vi "Instantaneous COR.vi"(1 "Data Input":T1 {"Data Channels" format="%.2f"}) -> (0 "Data Output":T1 {"Data Channels" format="%.2f"})   [LabVIEW 2013]
uses:
  <vilib>/Analysis/baseanly.llb/Real A x B.vi
  <vilib>/Analysis/baseanly.llb/Real Inverse Matrix.vi
  comm/fick-matrix/fick-matrix.lvlib
  <vilib>/Analysis/NI_AALBase.lvlib
panel:
  in  "Bite-piece channels":cluster{"List 1":u16, "Boolean 2":bool}[](array[cluster])=[{"List 1"=25, "Boolean 2"=TRUE}, {"List 1"=29, "Boolean 2"=FALSE}, {"List 1"=27, "Boolean 2"=FALSE}] {"List 1" items=["Hz Position-in-Head", "Hy Position-in-Head", "Hx Position-in-Head", "Hx Velocity-in-Head", "Hy Velocity-in-Head", "Hz Velocity-in-Head", "Hl Velocity-in-Head", "Hr Velocity-in-Head", "Lz Position-in-Head", "Ly Position-in-Head", "Lx Position-in-Head", "Lx Velocity-in-Head", "Ly Velocity-in-Head", "Lz Velocity-in-Head", "Ll Velocity-in-Head", "Lr Velocity-in-Head", "Rz Position-in-Head", "Ry Position-in-Head", "Rx Position-in-Head", "Rx Velocity-in-Head", "Ry Velocity-in-Head", "Rz Velocity-in-Head", "Rl Velocity-in-Head", "Rr Velocity-in-Head", "Button", "Ascension X", "Ascension X Vel", "Ascension Y", "Ascension Y Vel", "Ascension Z", "Chair Position", "Chair Velocity", " "]}
  in  "Head Channels":cluster{"List 1":u16, "Boolean 2":bool}[](array[cluster])=[{"List 1"=0, "Boolean 2"=FALSE}, {"List 1"=1, "Boolean 2"=FALSE}, {"List 1"=2, "Boolean 2"=FALSE}] {"List 1" items=["Hz Position-in-Head", "Hy Position-in-Head", "Hx Position-in-Head", "Hx Velocity-in-Head", "Hy Velocity-in-Head", "Hz Velocity-in-Head", "Hl Velocity-in-Head", "Hr Velocity-in-Head", "Lz Position-in-Head", "Ly Position-in-Head", "Lx Position-in-Head", "Lx Velocity-in-Head", "Ly Velocity-in-Head", "Lz Velocity-in-Head", "Ll Velocity-in-Head", "Lr Velocity-in-Head", "Rz Position-in-Head", "Ry Position-in-Head", "Rx Position-in-Head", "Rx Velocity-in-Head", "Ry Velocity-in-Head", "Rz Velocity-in-Head", "Rl Velocity-in-Head", "Rr Velocity-in-Head", "Button", "Ascension X", "Ascension X Vel", "Ascension Y", "Ascension Y Vel", "Ascension Z", "Chair Position", "Chair Velocity", " "]}
  # "Inv                 Channel"
  # "Head Z Fick position (deg)\n\nHead Y\n\nHead X"
  # "Inv                 Channel"
  # "Bite-piece X position (mm)\n\nBite-piece Y\n\nBite-piece Z"
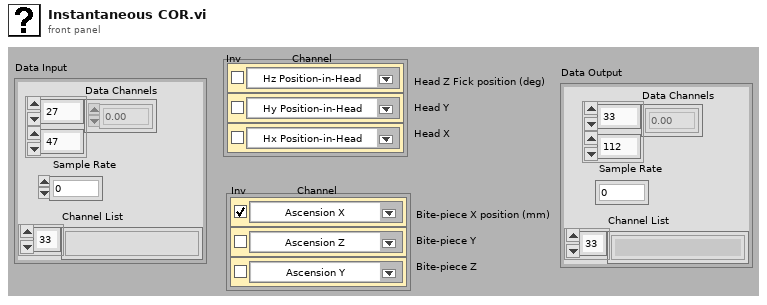
[diagram p1: front panel]
types:
  T1 = cluster{"Data Channels":dbl[][], "Sample Rate":i32, "Channel List":string[]}
  T2 = typedef "NI_Matrix.lvlib/RealMatrix.ctl" = dbl[][]
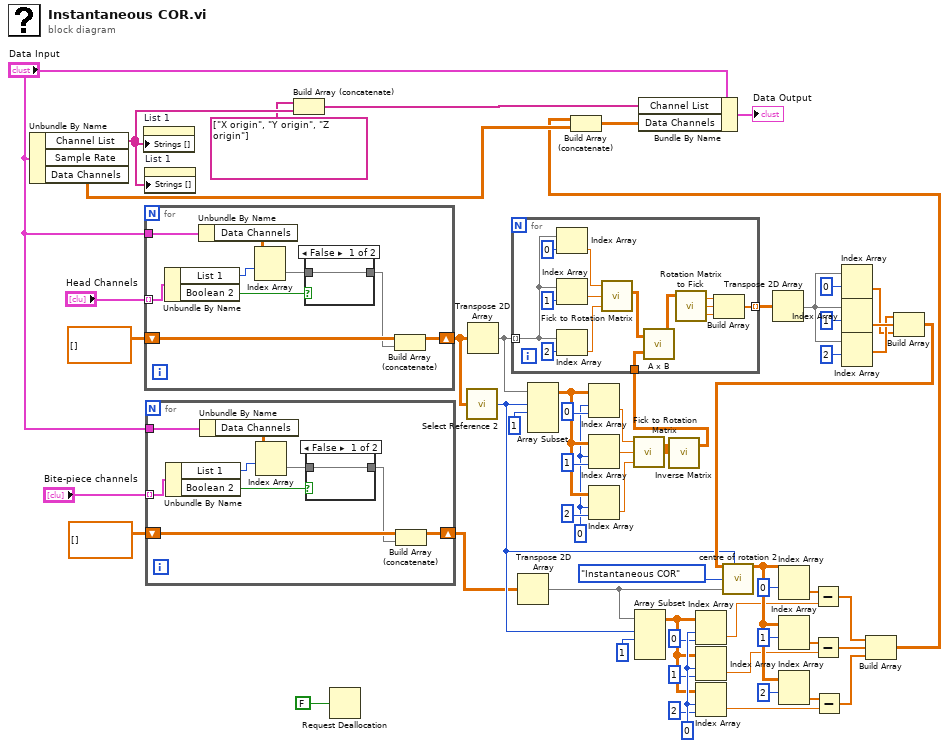
[diagram p0: block diagram]
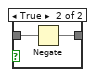
[diagram p2: hidden frame]
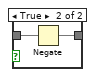
[diagram p3: hidden frame]
diagram:
  w13 = 0 ("disabled index (col)")
  w45 = 0 ("disabled index (col)")
  n1 = Unbundle By Name("Data Input") -> ("Channel List"=w34:string[], "Data Channels"=w35:dbl[][])  [unwired: 1 out]
  n2 = property on="List 1" class="Ring (strict)"("Strings []"=w34) -> ()  [unwired: 2 in, 2 out]
  n3 = property on="List 1" class="Ring (strict)"("Strings []"=w34) -> ()  [unwired: 2 in, 2 out]
  n4 = for {
    tunnel: "Head Channels" -> [w67] mode=indexing
    tunnel: "Data Input" -> [w64]
    shift-right: [w66] -> w37
    shift-left: dbl[][] [] -> [w65]
    n5 = Unbundle By Name(w67) -> ("List 1"=w62:u16, "Boolean 2"=w61:bool)
    n6 = Unbundle By Name(w64) -> ("Data Channels"=w63:dbl[][])
    n7 = Index Array(array=w63, index (row)=w62) -> (element=w60:dbl[])  [unwired: 1 in]
    n8 = case shown="False" w61 {
      tunnel: w60 -> [w68 w70]
      tunnel: [w68 w69] -> w59
      frame False {
      }
      frame True {
        n9 = Negate(x=w70) -> (-x=w69:dbl[])
      }
    }
    n10 = Build Array (concatenate)(w65, w59) -> (w66:dbl[][])
  }
  n11 = for {
    tunnel: "Bite-piece channels" -> [w79] mode=indexing
    tunnel: "Data Input" -> [w76]
    shift-right: [w78] -> w6
    shift-left: dbl[][] [] -> [w77]
    n12 = Unbundle By Name(w79) -> ("List 1"=w74:u16, "Boolean 2"=w73:bool)
    n13 = Unbundle By Name(w76) -> ("Data Channels"=w75:dbl[][])
    n14 = Index Array(array=w75, index (row)=w74) -> (element=w72:dbl[])  [unwired: 1 in]
    n15 = case shown="False" w73 {
      tunnel: w72 -> [w80 w82]
      tunnel: [w80 w81] -> w71
      frame False {
      }
      frame True {
        n16 = Negate(x=w82) -> (-x=w81:dbl[])
      }
    }
    n17 = Build Array (concatenate)(w77, w71) -> (w78:dbl[][])
  }
  n18 = Build Array (concatenate)(string[] ["X origin", "Y origin", "Z origin"], w34) -> (w40:string[])
  n19 = Request Deallocation(FALSE ("flag")) -> ()
  n20 = call "Select Reference 2.vi"("3D Coil"=w37) -> ("Element Data"=w7:i32)
  n21 = Transpose 2D Array(2D array=w37) -> (transposed array=w36:dbl[][])
  n22 = Transpose 2D Array(2D array=w6) -> (transposed array=w2:dbl[][])
  n23 = Array Subset(array=w36, index (row)=w7, length (row)=1 ("length")) -> (w53:dbl[][])  [unwired: 2 in]
  n24 = Index Array(array=w53, index (row)=w45, index (col)=0 ("index (row)")) -> (element=w52:dbl)
  n25 = Index Array(array=w53, index (row)=w45, index (col)=1 ("index (row)")) -> (element=w51:dbl)
  n26 = Index Array(array=w53, index (row)=w45, index (col)=2 ("index (row)")) -> (element=w50:dbl)
  n27 = call "Fick to Rotation Matrix.vi"("T"=w50, "V"=w51, "H"=w52) -> ("Rotation Matrix"=w49:dbl[][])
  n28 = Array Subset(array=w2, index (row)=w7, length (row)=1 ("length")) -> (w9:dbl[][])  [unwired: 2 in]
  n29 = call-poly <vilib>:"Inverse Matrix.vi"("Input Matrix"=w49) -> ("Inverse Matrix"=w44:T2)  [unwired: 1 in, 1 out]
  n30 = for {
    tunnel: w36 -> [w90] mode=indexing
    tunnel: w44 -> [w89]
    tunnel: [w83] -> w43 mode=indexing
    n31 = Index Array(array=w90, index=0 ("index (row)")) -> (element=w94:dbl)
    n32 = Index Array(array=w90, index=1 ("index (row)")) -> (element=w95:dbl)
    n33 = Index Array(array=w90, index=2 ("index (row)")) -> (element=w96:dbl)
    n34 = call "Fick to Rotation Matrix.vi"("T"=w96, "V"=w95, "H"=w94) -> ("Rotation Matrix"=w88:dbl[][])
    n35 = call-poly <vilib>:"A x B.vi"("B"=w89, "A"=w88) -> ("A x B"=w87:T2)  [unwired: 1 out]
    n36 = call "Rotation Matrix to Fick.vi"("A"=w87) -> ("T"=w84:dbl, "V"=w85:dbl, "H"=w86:dbl)  [unwired: 2 in]
    n37 = Build Array(w86, w85, w84) -> (w83:dbl[])
  }
  n38 = Index Array(array=w9, index (row)=w13, index (col)=0 ("index (row)")) -> (element=w5:dbl)
  n39 = Index Array(array=w9, index (row)=w13, index (col)=1 ("index (row)")) -> (element=w4:dbl)
  n40 = Index Array(array=w9, index (row)=w13, index (col)=2 ("index (row)")) -> (element=w3:dbl)
  n41 = Transpose 2D Array(2D array=w43) -> (transposed array=w21:dbl[][])
  n42 = Index Array(array=w21, index (row)=0) -> (element=w15:dbl[])  [unwired: 1 in]
  n43 = Index Array(array=w21, index (row)=1) -> (element=w17:dbl[])  [unwired: 1 in]
  n44 = Index Array(array=w21, index (row)=2) -> (element=w16:dbl[])  [unwired: 1 in]
  n45 = Build Array(w16, w17, w15) -> (w14:dbl[][])
  n46 = call "centre of rotation 2.vi"("Head rotation (Fick)"=w14, "reference"=w7, "Analysis"=enum16{"Instantaneous COR", "Average COR"}."Instantaneous COR", "POSITION 3D"=w2) -> ("Coefficients"=w32:dbl[][])  [unwired: 10 in, 1 out]
  n47 = Index Array(array=w32, index (row)=0) -> (element=w28:dbl[])  [unwired: 1 in]
  n48 = Index Array(array=w32, index (row)=1) -> (element=w27:dbl[])  [unwired: 1 in]
  n49 = Index Array(array=w32, index (row)=2) -> (element=w26:dbl[])  [unwired: 1 in]
  n50 = Subtract(x=w28, y=w5) -> (x-y=w23:dbl[])
  n51 = Subtract(x=w27, y=w4) -> (x-y=w25:dbl[])
  n52 = Subtract(x=w26, y=w3) -> (x-y=w24:dbl[])
  n53 = Build Array(w23, w25, w24) -> (w22:dbl[][])
  n54 = Build Array (concatenate)(w22, w35) -> (w39:dbl[][])
  n55 = Bundle By Name(cluster="Data Input", "Channel List"=w40, "Data Channels"=w39) -> (→"Data Output":T1)
